vi "Gaussian Filter(Pic1 Level2-4).vi"(0 "Cols":i16, 1 "Rows":i16, 2 "Width":u32, 3 "Height":u32, 5 "Data In":u8, 7 "DV In":bool, 9 "delayRowCount":i16, 12 "Memory In":refnum<k21>) -> (16 "DV out":bool, 17 "Data Out":fxp<+,12,12>)   [LabVIEW 2016]
uses:
  <vilib>/rvi/DataTransferAndStorage/Container/Common/niFpgaContainerExecOnDevCompGetState.vi
  <vilib>/rvi/Emulation/niFpgaEmulationIsFPGAContextNoSignature.vi
  <vilib>/rvi/DataTransferAndStorage/Container/Common/niFpgaContainerGetUniqueNameForEmu.vi
  <vilib>/rvi/Emulation/niFpgaProcessEmulError.vi
  <vilib>/rvi/Emulation/niFpgaSctlEmulationGetInTimedLoop.vi
  <vilib>/rvi/errors/nirviReportUnexpectedCaseInternalError (U32).vi
  <vilib>/rvi/Memory/Memory_Emulation/niFpgaMemoryEmulationCacheClearOnFirstRun.vi
  <vilib>/rvi/Memory/Memory_Emulation/nirvimemoryEmulationManagerCache_MakeExclusive.vi
  <vilib>/rvi/Memory/Memory_Emulation/niFpgaMemoryEmulationValidateCache.vi
  <vilib>/rvi/Memory/Memory_Emulation/nirvimemoryEmulationManagerCache_InsertValue.vi
  <vilib>/Utility/error.llb/Clear Errors.vi
  <vilib>/rvi/Memory/Memory_Emulation/nirvimemoryEmulationManagerCache_ReleaseExclusive.vi
  <vilib>/rvi/Memory/Memory_Emulation/nirvimemoryEmulationManagerCache_GetValue.vi
  <vilib>/rvi/Memory/Memory_Emulation/nirvimemoryEmulationManagerCache_SetValue.vi
  <vilib>/rvi/Emulation/niFpgaSctlEmulationResourceMgr.vi
  <vilib>/rvi/DataTransferAndStorage/Container/XNode/niFpgaContainer.xnode
  <vilib>/rvi/Memory/Memory_Emulation/niFpgaMemoryEmulationRefIn.vi
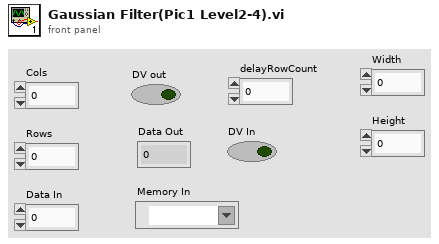
[diagram p1: front panel]
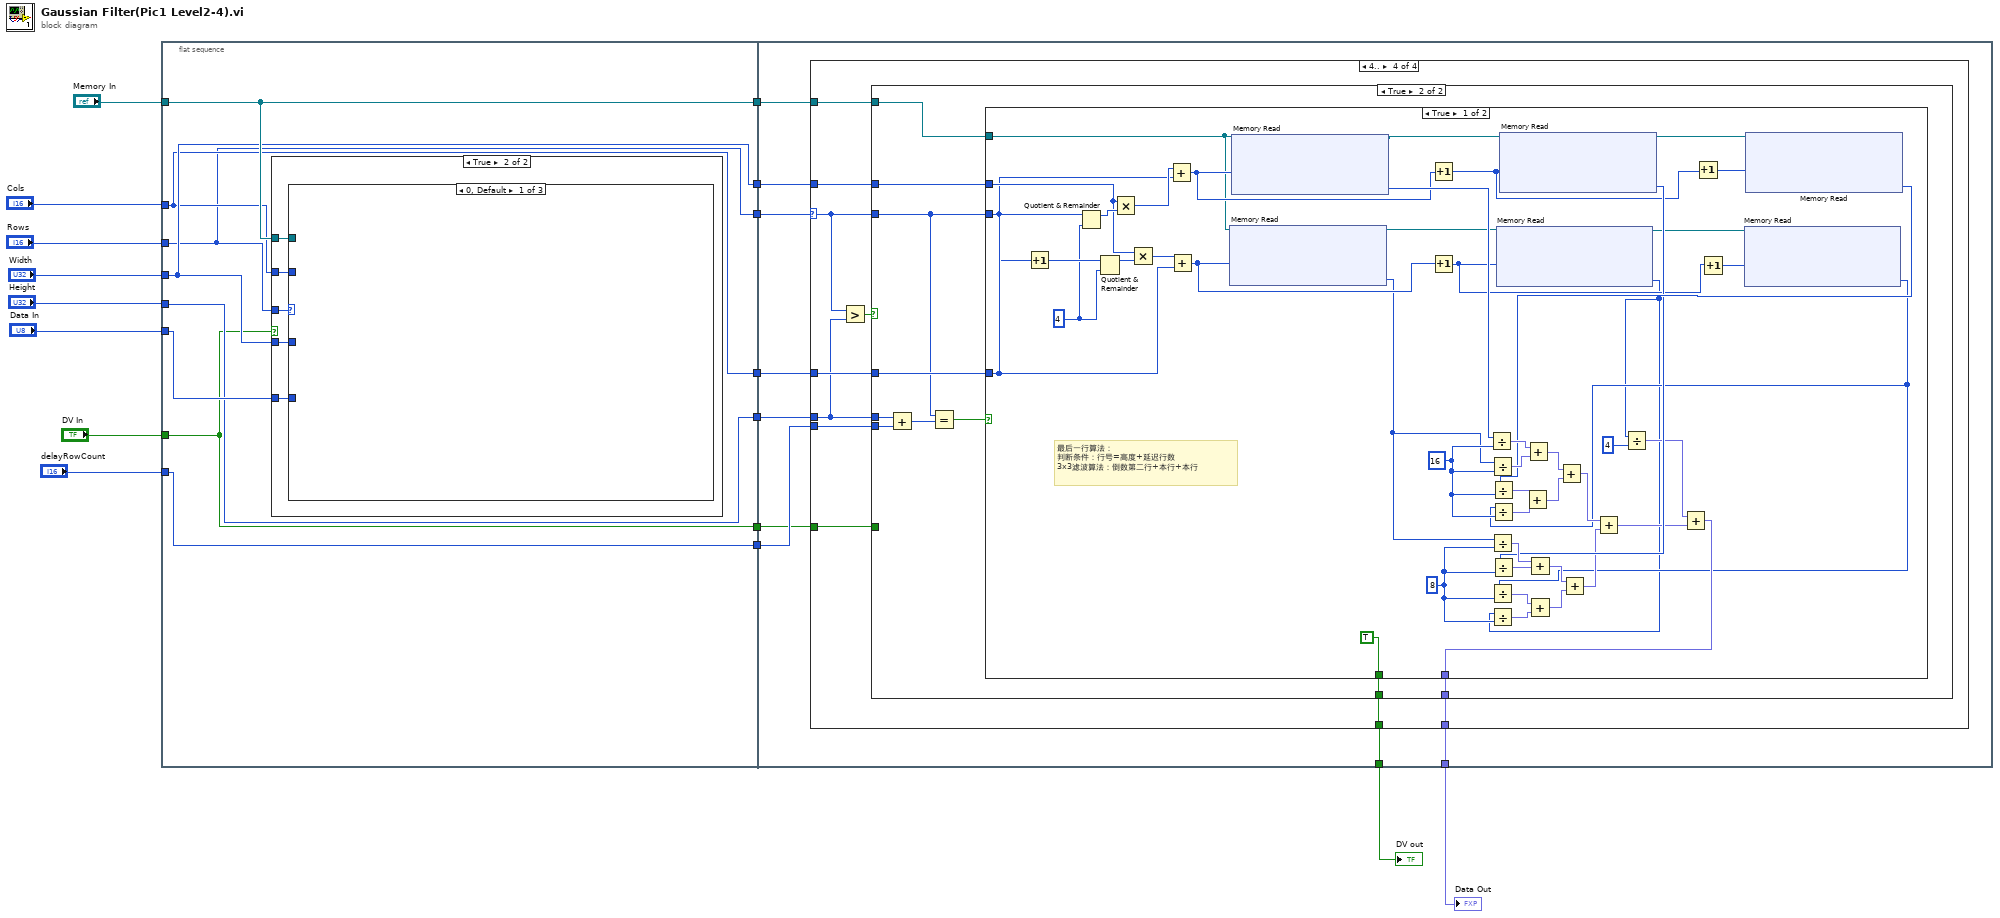
[diagram p0: block diagram]
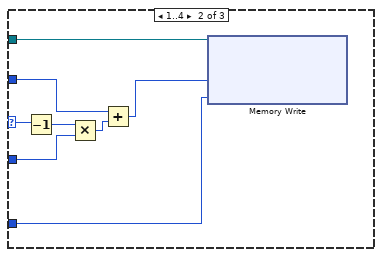
[diagram p3: hidden frame]
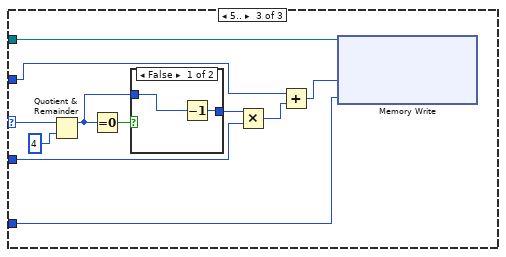
[diagram p4: hidden frame]
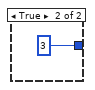
[diagram p5: hidden frame]
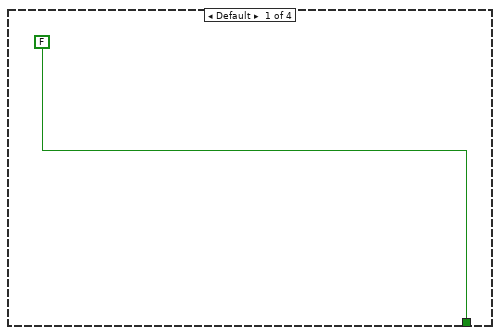
[diagram p6: hidden frame]
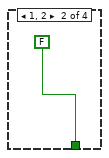
[diagram p7: hidden frame]
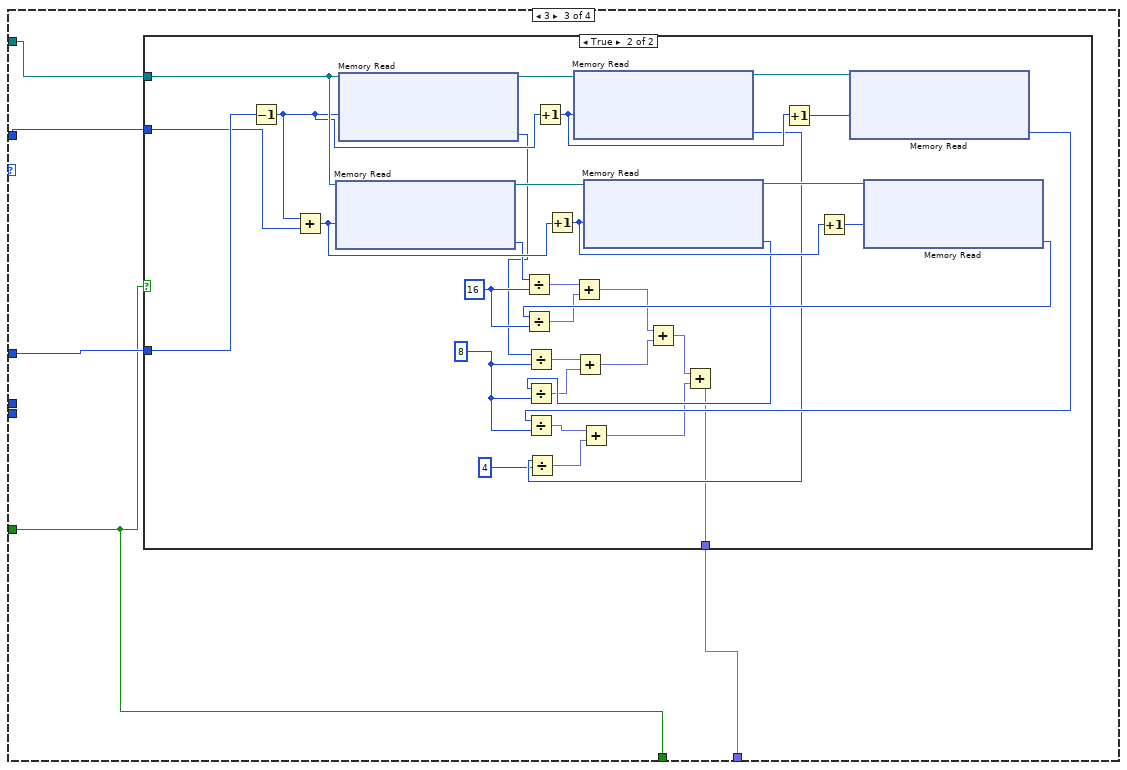
[diagram p8: hidden frame]
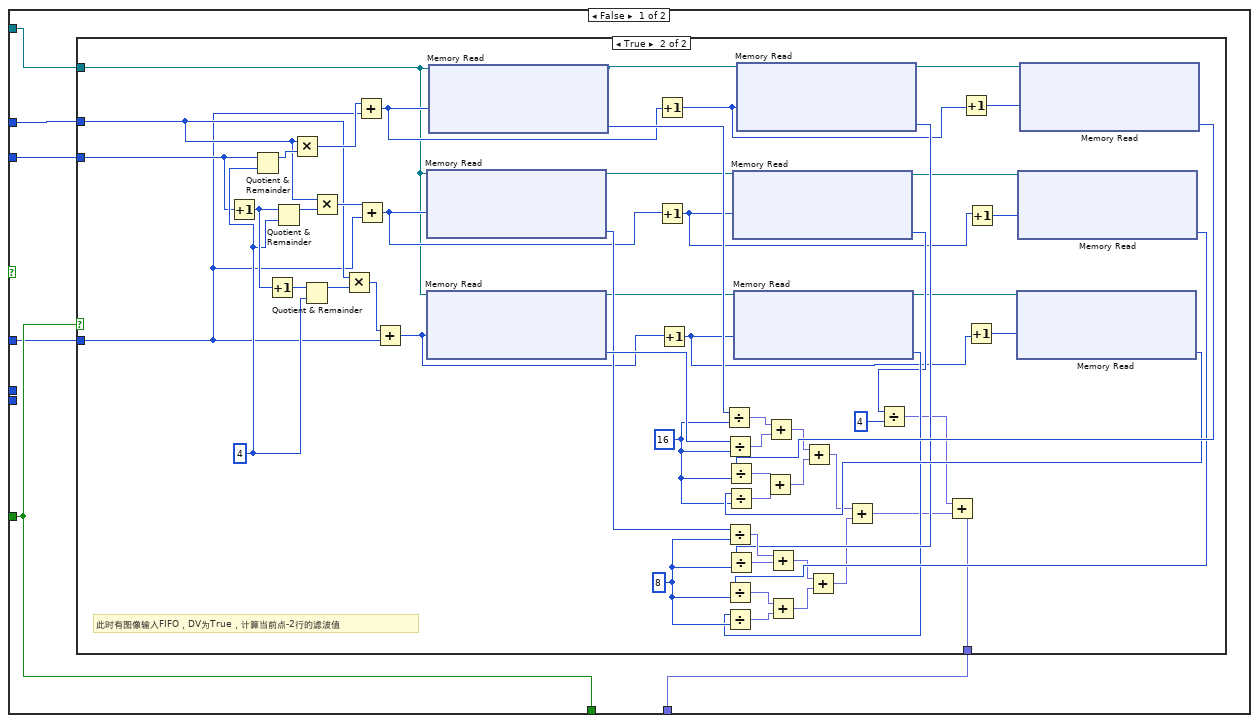
[diagram p10: hidden frame]
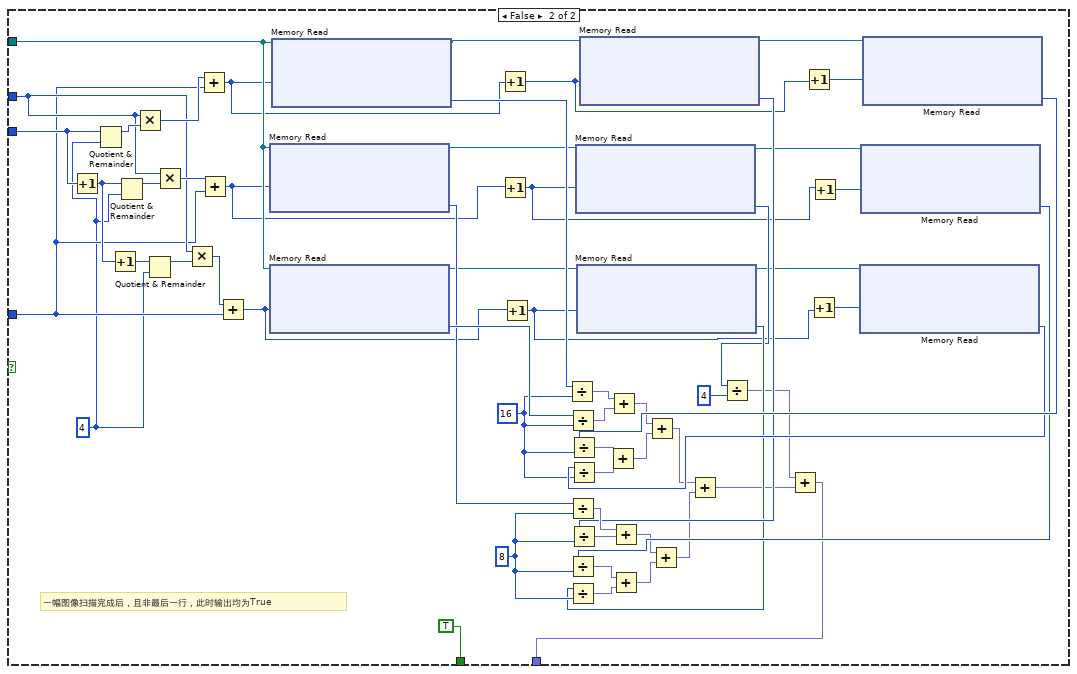
[diagram p12: hidden frame]
diagram:
  n1 = flat-sequence {
    tunnel: [w21] -> w17
    tunnel: [w23] -> w16
    tunnel: [w22] -> w15
    tunnel: [w24] -> w14
    tunnel: [w18] -> w13
    tunnel: [w20] -> w12
    tunnel: [w19] -> w11
    tunnel: "Rows" -> [w21]
    tunnel: "Memory In" -> [w24]
    tunnel: "Cols" -> [w22]
    tunnel: "Data In" -> [w25]
    tunnel: "Width" -> [w23]
    tunnel: "Height" -> [w20]
    tunnel: "DV In" -> [w19]
    tunnel: "delayRowCount" -> [w18]
    tunnel: w17 -> [w61]
    tunnel: w16 -> [w58]
    tunnel: w15 -> [w59]
    tunnel: w14 -> [w60]
    tunnel: [w57] -> w3
    tunnel: [w56] -> w4
    tunnel: w13 -> [w55]
    tunnel: w12 -> [w54]
    tunnel: w11 -> [w53]
    frame #0 {
      n2 = case shown="True" w19 {
        tunnel: w25 -> [_ w30]
        tunnel: w21 -> [_ w29]
        tunnel: w23 -> [_ w28]
        tunnel: w22 -> [_ w27]
        tunnel: w24 -> [_ w26]
        frame False {
        }
        frame True {
          n3 = case shown="0, Default" w29 {
            selector: w29 -> [_ w37 w49]
            tunnel: w26 -> [_ w38 w41]
            tunnel: w27 -> [_ w33 w42]
            tunnel: w30 -> [_ w31 w39]
            tunnel: w28 -> [_ w35 w44]
            frame 0, Default {
            }
            frame 1..4 {
              n4 = Decrement(x=w37) -> (x-1=w36:i16)
              n5 = Multiply(x=w36, y=w35) -> (x*y=w34:u32)
              n6 = Add(x=w33, y=w34) -> (x+y=w32:u32)
              n7 = xnode ("Memory Write")("Address"=w32, "Data"=w31, "Memory In"=w38) -> ()  [unwired: 1 out]
            }
            frame 5.. {
              n8 = Quotient & Remainder(x=w49, y=i16 4) -> (x-y*floor(x/y)=w46:i16)  [unwired: 1 out]
              n9 = Equal To 0?(x=w46) -> (x = 0?=w47:bool)
              n10 = case shown="False" w47 {
                tunnel: w46 -> [w50 _]
                tunnel: [w51 i16 3] -> w45
                frame False {
                  n11 = Decrement(x=w50) -> (x-1=w51:i16)
                }
                frame True {
                }
              }
              n12 = Multiply(x=w45, y=w44) -> (x*y=w43:u32)
              n13 = Add(x=w42, y=w43) -> (x+y=w40:u32)
              n14 = xnode ("Memory Write")("Address"=w40, "Data"=w39, "Memory In"=w41) -> ()  [unwired: 1 out]
            }
          }
        }
      }
    }
    frame #1 {
      n15 = case shown="4.." w61 {
        selector: w61 -> [_ _ _ w104]
        tunnel: w60 -> [_ _ w68 w111]
        tunnel: w59 -> [_ _ w67 w107]
        tunnel: w58 -> [_ _ w66 w108]
        tunnel: [_ _ w65 w110] -> w57
        tunnel: [FALSE FALSE w64 w109] -> w56
        tunnel: w55 -> [_ _ _ w106]
        tunnel: w54 -> [_ _ _ w103]
        tunnel: w53 -> [_ _ w64 w102]
        frame Default {
        }
        frame 1, 2 {
        }
        frame 3 {
          n16 = case shown="True" w64 {
            tunnel: w68 -> [_ w98]
            tunnel: w67 -> [_ w96]
            tunnel: w66 -> [_ w95]
            tunnel: [_ w69] -> w65
            frame False {
            }
            frame True {
              w82 = u8 8 ("y")
              w87 = u8 16 ("y")
              n17 = Decrement(x=w96) -> (x-1=w92:i16)
              n18 = Add(x=w92, y=w95) -> (x+y=w93:u32)
              n19 = xnode "Memory Read"("Address"=w93, "Memory In"=w98) -> ("Data"=w88:u8, "Memory Out"=w97:refnum<k21>)
              n20 = xnode "Memory Read"("Address"=w92, "Memory In"=w98) -> ("Data"=w83:u8, "Memory Out"=w101:refnum<k21>)
              n21 = Divide(x=w88, y=w87) -> (x/y=w85:fxp<+,8,8>)
              n22 = Divide(x=w83, y=w82) -> (x/y=w77:fxp<+,8,8>)
              n23 = Increment(x=w92) -> (x+1=w90:i16)
              n24 = Increment(x=w93) -> (x+1=w89:u32)
              n25 = xnode "Memory Read"("Address"=w90, "Memory In"=w101) -> ("Data"=w79:u8, "Memory Out"=w100:refnum<k21>)
              n26 = Divide(x=w79, y=u8 4) -> (x/y=w74:fxp<+,8,8>)
              n27 = xnode "Memory Read"("Address"=w89, "Memory In"=w97) -> ("Data"=w81:u8, "Memory Out"=w94:refnum<k21>)
              n28 = Divide(x=w81, y=w82) -> (x/y=w76:fxp<+,8,8>)
              n29 = Add(x=w77, y=w76) -> (x+y=w72:fxp<+,9,9>)
              n30 = Increment(x=w90) -> (x+1=w99:i16)
              n31 = Increment(x=w89) -> (x+1=w91:u32)
              n32 = xnode "Memory Read"("Address"=w99, "Memory In"=w100) -> ("Data"=w80:u8)  [unwired: 1 out]
              n33 = Divide(x=w80, y=w82) -> (x/y=w75:fxp<+,8,8>)
              n34 = Add(x=w75, y=w74) -> (x+y=w70:fxp<+,9,9>)
              n35 = xnode "Memory Read"("Address"=w91, "Memory In"=w94) -> ("Data"=w86:u8)  [unwired: 1 out]
              n36 = Divide(x=w86, y=w87) -> (x/y=w84:fxp<+,8,8>)
              n37 = Add(x=w85, y=w84) -> (x+y=w73:fxp<+,9,9>)
              n38 = Add(x=w73, y=w72) -> (x+y=w71:fxp<+,10,10>)
              n39 = Add(x=w71, y=w70) -> (x+y=w69:fxp<+,11,11>)
            }
          }
        }
        frame 4.. {
          n40 = Greater?(x=w104, y=w103) -> (0:w105:bool)
          n41 = case shown="True" w105 {
            tunnel: w111 -> [w114 w184]
            tunnel: [w116 w183] -> w110
            tunnel: [w117 w182] -> w109
            tunnel: w108 -> [w113 w181]
            tunnel: w107 -> [w112 w180]
            tunnel: w106 -> [_ w179]
            tunnel: w103 -> [_ w178]
            tunnel: w104 -> [w115 w176]
            tunnel: w102 -> [w117 _]
            frame False {
              n42 = case shown="True" w117 {
                tunnel: [_ w122] -> w116
                tunnel: w115 -> [_ w121]
                tunnel: w114 -> [_ w120]
                tunnel: w113 -> [_ w119]
                tunnel: w112 -> [_ w118]
                frame False {
                  # "此时输入FIFO有图像输入，DV为False，不输出结果"
                }
                frame True {
                  w123 = u32 4 ("y")
                  w161 = u8 8 ("y")
                  w164 = u8 16 ("y")
                  # "此时有图像输入FIFO，DV为True，计算当前点-2行的滤波值"
                  n43 = Increment(x=w121) -> (x+1=w128:i16)
                  n44 = Quotient & Remainder(x=w121, y=w123) -> (x-y*floor(x/y)=w140:u32)  [unwired: 1 out]
                  n45 = Increment(x=w128) -> (x+1=w127:i16)
                  n46 = Quotient & Remainder(x=w128, y=w123) -> (x-y*floor(x/y)=w126:u32)  [unwired: 1 out]
                  n47 = Multiply(x=w119, y=w140) -> (x*y=w139:u32)
                  n48 = Quotient & Remainder(x=w127, y=w123) -> (x-y*floor(x/y)=w125:u32)  [unwired: 1 out]
                  n49 = Multiply(x=w119, y=w126) -> (x*y=w129:u32)
                  n50 = Multiply(x=w119, y=w125) -> (x*y=w124:u32)
                  n51 = Add(x=w139, y=w118) -> (x+y=w136:u32)
                  n52 = Add(x=w129, y=w118) -> (x+y=w133:u32)
                  n53 = Add(x=w124, y=w118) -> (x+y=w132:u32)
                  n54 = xnode "Memory Read"("Address"=w133, "Memory In"=w120) -> ("Data"=w160:u8, "Memory Out"=w144:refnum<k21>)
                  n55 = xnode "Memory Read"("Address"=w132, "Memory In"=w120) -> ("Data"=w173:u8, "Memory Out"=w142:refnum<k21>)
                  n56 = xnode "Memory Read"("Address"=w136, "Memory In"=w120) -> ("Data"=w174:u8, "Memory Out"=w146:refnum<k21>)
                  n57 = Increment(x=w136) -> (x+1=w137:u32)
                  n58 = Increment(x=w133) -> (x+1=w134:u32)
                  n59 = Increment(x=w132) -> (x+1=w130:u32)
                  n60 = Divide(x=w174, y=w164) -> (x/y=w172:fxp<+,8,8>)
                  n61 = Divide(x=w173, y=w164) -> (x/y=w171:fxp<+,8,8>)
                  n62 = Divide(x=w160, y=w161) -> (x/y=w163:fxp<+,8,8>)
                  n63 = xnode "Memory Read"("Address"=w134, "Memory In"=w144) -> ("Data"=w156:u8, "Memory Out"=w143:refnum<k21>)
                  n64 = xnode "Memory Read"("Address"=w130, "Memory In"=w142) -> ("Data"=w157:u8, "Memory Out"=w141:refnum<k21>)
                  n65 = Divide(x=w157, y=w161) -> (x/y=w165:fxp<+,8,8>)
                  n66 = xnode "Memory Read"("Address"=w137, "Memory In"=w146) -> ("Data"=w159:u8, "Memory Out"=w145:refnum<k21>)
                  n67 = Divide(x=w159, y=w161) -> (x/y=w162:fxp<+,8,8>)
                  n68 = Add(x=w172, y=w171) -> (x+y=w150:fxp<+,9,9>)
                  n69 = Add(x=w163, y=w162) -> (x+y=w148:fxp<+,9,9>)
                  n70 = Divide(x=w156, y=u8 4) -> (x/y=w152:fxp<+,8,8>)
                  n71 = Increment(x=w137) -> (x+1=w138:u32)
                  n72 = Increment(x=w130) -> (x+1=w131:u32)
                  n73 = Increment(x=w134) -> (x+1=w135:u32)
                  n74 = xnode "Memory Read"("Address"=w131, "Memory In"=w141) -> ("Data"=w167:u8)  [unwired: 1 out]
                  n75 = Divide(x=w167, y=w164) -> (x/y=w169:fxp<+,8,8>)
                  n76 = xnode "Memory Read"("Address"=w135, "Memory In"=w143) -> ("Data"=w158:u8)  [unwired: 1 out]
                  n77 = Divide(x=w158, y=w161) -> (x/y=w166:fxp<+,8,8>)
                  n78 = Add(x=w166, y=w165) -> (x+y=w147:fxp<+,9,9>)
                  n79 = Add(x=w148, y=w147) -> (x+y=w153:fxp<+,10,10>)
                  n80 = xnode "Memory Read"("Address"=w138, "Memory In"=w145) -> ("Data"=w168:u8)  [unwired: 1 out]
                  n81 = Divide(x=w168, y=w164) -> (x/y=w170:fxp<+,8,8>)
                  n82 = Add(x=w170, y=w169) -> (x+y=w149:fxp<+,9,9>)
                  n83 = Add(x=w150, y=w149) -> (x+y=w154:fxp<+,10,10>)
                  n84 = Add(x=w154, y=w153) -> (x+y=w151:fxp<+,11,11>)
                  n85 = Add(x=w152, y=w151) -> (x+y=w122:fxp<+,12,12>)
                }
              }
            }
            frame True {
              n86 = Add(x=w178, y=w179) -> (x+y=w177:u32)
              n87 = Equal?(x=w176, y=w177) -> (x = y?=w175:bool)
              n88 = case shown="True" w175 {
                tunnel: w184 -> [w193 w257]
                tunnel: [w188 w254] -> w183
                tunnel: [TRUE TRUE] -> w182
                tunnel: w176 -> [w190 w241]
                tunnel: w181 -> [w192 w235]
                tunnel: w180 -> [w191 w233]
                frame True {
                  w194 = u32 4 ("y")
                  w220 = u8 8 ("y")
                  w223 = u8 16 ("y")
                  # "最后一行算法：\n判断条件：行号=高度+延迟行数\n3x3滤波算法：倒数第二行+本行+本行"
                  n89 = Increment(x=w190) -> (x+1=w196:i16)
                  n90 = Quotient & Remainder(x=w190, y=w194) -> (x-y*floor(x/y)=w205:u32)  [unwired: 1 out]
                  n91 = Quotient & Remainder(x=w196, y=w194) -> (x-y*floor(x/y)=w195:u32)  [unwired: 1 out]
                  n92 = Multiply(x=w192, y=w205) -> (x*y=w204:u32)
                  n93 = Multiply(x=w192, y=w195) -> (x*y=w197:u32)
                  n94 = Add(x=w204, y=w191) -> (x+y=w201:u32)
                  n95 = Add(x=w197, y=w191) -> (x+y=w198:u32)
                  n96 = xnode "Memory Read"("Address"=w198, "Memory In"=w193) -> ("Data"=w187:u8, "Memory Out"=w207:refnum<k21>)
                  n97 = xnode "Memory Read"("Address"=w201, "Memory In"=w193) -> ("Data"=w231:u8, "Memory Out"=w209:refnum<k21>)
                  n98 = Increment(x=w201) -> (x+1=w202:u32)
                  n99 = Increment(x=w198) -> (x+1=w199:u32)
                  n100 = Divide(x=w231, y=w223) -> (x/y=w230:fxp<+,8,8>)
                  n101 = Divide(x=w187, y=w223) -> (x/y=w229:fxp<+,8,8>)
                  n102 = Divide(x=w187, y=w220) -> (x/y=w222:fxp<+,8,8>)
                  n103 = xnode "Memory Read"("Address"=w199, "Memory In"=w207) -> ("Data"=w185:u8, "Memory Out"=w206:refnum<k21>)
                  n104 = Divide(x=w185, y=w220) -> (x/y=w224:fxp<+,8,8>)
                  n105 = xnode "Memory Read"("Address"=w202, "Memory In"=w209) -> ("Data"=w219:u8, "Memory Out"=w208:refnum<k21>)
                  n106 = Divide(x=w219, y=w220) -> (x/y=w221:fxp<+,8,8>)
                  n107 = Add(x=w230, y=w229) -> (x+y=w213:fxp<+,9,9>)
                  n108 = Add(x=w222, y=w221) -> (x+y=w211:fxp<+,9,9>)
                  n109 = Divide(x=w185, y=u8 4) -> (x/y=w215:fxp<+,8,8>)
                  n110 = Increment(x=w202) -> (x+1=w203:u32)
                  n111 = Increment(x=w199) -> (x+1=w200:u32)
                  n112 = xnode "Memory Read"("Address"=w200, "Memory In"=w206) -> ("Data"=w186:u8)  [unwired: 1 out]
                  n113 = Divide(x=w186, y=w220) -> (x/y=w225:fxp<+,8,8>)
                  n114 = Divide(x=w186, y=w223) -> (x/y=w227:fxp<+,8,8>)
                  n115 = Add(x=w225, y=w224) -> (x+y=w210:fxp<+,9,9>)
                  n116 = Add(x=w211, y=w210) -> (x+y=w216:fxp<+,10,10>)
                  n117 = xnode "Memory Read"("Address"=w203, "Memory In"=w208) -> ("Data"=w226:u8)  [unwired: 1 out]
                  n118 = Divide(x=w226, y=w223) -> (x/y=w228:fxp<+,8,8>)
                  n119 = Add(x=w228, y=w227) -> (x+y=w212:fxp<+,9,9>)
                  n120 = Add(x=w213, y=w212) -> (x+y=w217:fxp<+,10,10>)
                  n121 = Add(x=w217, y=w216) -> (x+y=w214:fxp<+,11,11>)
                  n122 = Add(x=w215, y=w214) -> (x+y=w188:fxp<+,12,12>)
                }
                frame False {
                  w232 = u32 4 ("y")
                  w276 = u8 8 ("y")
                  w279 = u8 16 ("y")
                  # "一幅图像扫描完成后，且非最后一行，此时输出均为True"
                  n123 = Increment(x=w241) -> (x+1=w239:i16)
                  n124 = Quotient & Remainder(x=w241, y=w232) -> (x-y*floor(x/y)=w252:u32)  [unwired: 1 out]
                  n125 = Increment(x=w239) -> (x+1=w238:i16)
                  n126 = Quotient & Remainder(x=w239, y=w232) -> (x-y*floor(x/y)=w237:u32)  [unwired: 1 out]
                  n127 = Multiply(x=w235, y=w252) -> (x*y=w251:u32)
                  n128 = Quotient & Remainder(x=w238, y=w232) -> (x-y*floor(x/y)=w236:u32)  [unwired: 1 out]
                  n129 = Multiply(x=w235, y=w237) -> (x*y=w240:u32)
                  n130 = Multiply(x=w235, y=w236) -> (x*y=w234:u32)
                  n131 = Add(x=w251, y=w233) -> (x+y=w248:u32)
                  n132 = Add(x=w240, y=w233) -> (x+y=w245:u32)
                  n133 = Add(x=w234, y=w233) -> (x+y=w244:u32)
                  n134 = xnode "Memory Read"("Address"=w245, "Memory In"=w257) -> ("Data"=w275:u8, "Memory Out"=w259:refnum<k21>)
                  n135 = xnode "Memory Read"("Address"=w244, "Memory In"=w257) -> ("Data"=w288:u8, "Memory Out"=w256:refnum<k21>)
                  n136 = xnode "Memory Read"("Address"=w248, "Memory In"=w257) -> ("Data"=w289:u8, "Memory Out"=w261:refnum<k21>)
                  n137 = Increment(x=w248) -> (x+1=w249:u32)
                  n138 = Increment(x=w245) -> (x+1=w246:u32)
                  n139 = Increment(x=w244) -> (x+1=w242:u32)
                  n140 = Divide(x=w289, y=w279) -> (x/y=w287:fxp<+,8,8>)
                  n141 = Divide(x=w288, y=w279) -> (x/y=w286:fxp<+,8,8>)
                  n142 = Divide(x=w275, y=w276) -> (x/y=w278:fxp<+,8,8>)
                  n143 = xnode "Memory Read"("Address"=w246, "Memory In"=w259) -> ("Data"=w271:u8, "Memory Out"=w258:refnum<k21>)
                  n144 = xnode "Memory Read"("Address"=w242, "Memory In"=w256) -> ("Data"=w272:u8, "Memory Out"=w255:refnum<k21>)
                  n145 = Divide(x=w272, y=w276) -> (x/y=w280:fxp<+,8,8>)
                  n146 = xnode "Memory Read"("Address"=w249, "Memory In"=w261) -> ("Data"=w274:u8, "Memory Out"=w260:refnum<k21>)
                  n147 = Divide(x=w274, y=w276) -> (x/y=w277:fxp<+,8,8>)
                  n148 = Add(x=w287, y=w286) -> (x+y=w265:fxp<+,9,9>)
                  n149 = Add(x=w278, y=w277) -> (x+y=w263:fxp<+,9,9>)
                  n150 = Divide(x=w271, y=u8 4) -> (x/y=w267:fxp<+,8,8>)
                  n151 = Increment(x=w249) -> (x+1=w250:u32)
                  n152 = Increment(x=w242) -> (x+1=w243:u32)
                  n153 = Increment(x=w246) -> (x+1=w247:u32)
                  n154 = xnode "Memory Read"("Address"=w243, "Memory In"=w255) -> ("Data"=w282:u8)  [unwired: 1 out]
                  n155 = Divide(x=w282, y=w279) -> (x/y=w284:fxp<+,8,8>)
                  n156 = xnode "Memory Read"("Address"=w247, "Memory In"=w258) -> ("Data"=w273:u8)  [unwired: 1 out]
                  n157 = Divide(x=w273, y=w276) -> (x/y=w281:fxp<+,8,8>)
                  n158 = Add(x=w281, y=w280) -> (x+y=w262:fxp<+,9,9>)
                  n159 = Add(x=w263, y=w262) -> (x+y=w268:fxp<+,10,10>)
                  n160 = xnode "Memory Read"("Address"=w250, "Memory In"=w260) -> ("Data"=w283:u8)  [unwired: 1 out]
                  n161 = Divide(x=w283, y=w279) -> (x/y=w285:fxp<+,8,8>)
                  n162 = Add(x=w285, y=w284) -> (x+y=w264:fxp<+,9,9>)
                  n163 = Add(x=w265, y=w264) -> (x+y=w269:fxp<+,10,10>)
                  n164 = Add(x=w269, y=w268) -> (x+y=w266:fxp<+,11,11>)
                  n165 = Add(x=w267, y=w266) -> (x+y=w254:fxp<+,12,12>)
                }
              }
            }
          }
        }
      }
    }
  }
  "DV out" <- w4
  "Data Out" <- w3
